vi "commander4.vi"() -> ()   [LabVIEW 2015]
uses:
  G_SEN.vi
  G_NAV.vi
  G_LCM.vi
  G_VEH.vi
  <vilib>/Analysis/Matrix/Numeric/Conversions/Array To Matrix - RA.vi
  <vilib>/Analysis/Matrix/Numeric/Conversions/Array To Matrix - RA2.vi
  <vilib>/Analysis/Matrix/Numeric/Multiply/Multiply - RM,RM.vi
  <vilib>/Analysis/Matrix/Numeric/Conversions/Matrix To Array - RM.vi
  G_PATH.vi
  G_DATA.vi
  <vilib>/Analysis/Matrix/NI_Matrix.lvlib
panel:
  in  "lpf gain":dbl=0.01 format="%#_13g"
  in  "KR":dbl
  in  "Kheading":dbl
  in  "Kdist":dbl
  out "String":string
  out "Taxi":dbl[](array[numeric])
  out "EURECAR_VISION":T1
  out "count":i32
  out "Array 3":picture[](array[picture])
  out "Array 2":picture[](array[picture])
  out "sign 2":picture[](array[picture])
  out "sign":picture[](array[picture])
  in  "TTL":bool
  out "STOP":bool
  out "go":bool
  in  "Steering gain":dbl=1.07
  in  "Steering LPF gain":dbl
  in  "vehicel width":dbl=2.1999999999999997
  out "obs shift":dbl=-0.0 format="%.2f"
  in  "lane keep":bool
  in  "vel":bool
  in  "replay":bool
  in  "lane":bool
  in  "x":dbl min=-5.0 max=5.0 step=1.0
  out "lane_shift":dbl
  in  "Shift LPF gain":dbl=0.95
  out "display":u32=20
  out "control":u32=10
  out "update":bool=TRUE
  in  "save lcm":bool
  out "LCM Recv Data":string="SDT_GPS_DATA\t550\rGGA_1\t275\rGGA_2\t275\rRMC_1\t275\rIBEO_2202_T\t686\rRMC_2\t275\rEYE_RAW_T\t549\rPOS_T\t5352\rPATH_T\t1373\rCAN_T\t5486\rCON_T\t5458\r"
  out "GPS DATA 2":T2={"type"="WAAS", "x_lcc"=-423.72650605501394, "y_lcc"=-797.2504532505071, "latdev"=0.92, "londev"=0.92, "sats"=11, "gps_l1_ranges"=0, "gps_l1_mask_ranges"=0, "gps_l2_mask_ranges"=0, "Heading"=152.5234544430902, "lon"=127.356186, "lat"=36.368267, "time"="01:10:55.0", "hgps"=151.67000000000002, "lag"=0.0, "MAP"="KAIST"} {"lag" format="%#_5g"; "hgps" format="%#_5g"; "lat" format="%#_11g"; "lon" format="%#_11g"; "Heading" format="%#_5g"; "latdev" format="%#_4g"; "londev" format="%#_4g"}
  in  "Obs":bool=TRUE
  in  "Log":bool
  out "path":u32=10
  out "sensor":u32=10 format="%02.0f"
  out "Speed limit":dbl=20.0
  out "collision":bool
  in  "Load WPT":bool
  in  "Max. Vel.":dbl=20.0 min=-5.0 max=120.0 step=5.0
  in  "RESET PATH":bool
  out "col":i16(graph)
  out "stop":bool
  in  "Reverse":bool
  in  "STOP":bool
  out "Waveform Chart 4":cluster{"auto":i16, "run":i16}(graph)={"auto"=1, "run"=0}
  out "Waveform Chart 3":T3(graph)={"Steer_input"=0.0, "Steer_output"=-2.5, "handle"=1.691462017818249}
  out "Waveform Chart 2":T4(graph)={"VS_des"=0.0, "VS_can"=30.952437500000002, "VS_des"=20.0}
  out "Heading":cluster{"Heading":dbl, "hgps":dbl}(graph)={"Heading"=152.5234544430902, "hgps"=151.67000000000002}
  out "XY Graph 2":cluster{"Y":dbl[], "Y":dbl[]}[](graph)=[{"Y"=[-423.72650605501394], "Y"=[-797.2504532505071]}, {"Y"=array[29568 elements], "Y"=array[29568 elements]}, {"Y"=array[29568 elements], "Y"=array[29568 elements]}, {"Y"=[-419.18788283563754], "Y"=[-805.7085038383482]}]
  out "Gauge":cluster{dbl, dbl, dbl}(knob)={0.0, 30.952437500000002, 20.0} scale=-20.0..140.0
  out "Meter":cluster{dbl, dbl, dbl}(knob)={0.0, -2.5, 1.691462017818249} scale=-550.0..550.0
  out "XY Graph":cluster{"Y":dbl[], "Y":dbl[]}[](graph)=[{"Y"=[0.0], "Y"=[0.0]}, {"Y"=array[500 elements], "Y"=array[500 elements]}, {"Y"=array[500 elements], "Y"=array[500 elements]}, {"Y"=[], "Y"=[]}, {"Y"=[-0.003264064170771075], "Y"=[-0.9807019516255565]}, {"Y"=[], "Y"=[]}, {"Y"=[0.0, 3.415667538320122e-05, 0.00013662669994118914, 0.00030741006844436924, 0.0005465067717977945, 0.0008539167977232864, 0.0012296401303046878, 0.0016736767499878624, 0.002186026633808069, 0.002766689755162588, 0.0034156660840380937, 0.004132955586555909, 0.0049185582258814975, 0.005772473960860225, 0.006694702747381598, 0.007685244537924518, 0.008744099280875162, 0.009871266920981725, 0.011066747400491295, 0.01233054065687611, 0.013662646624879926, 0.015063065235381146, 0.016531796415847566, 0.01806884008965426, 0.019674196177675185, 0.021347864596464206, 0.023089845258937203, 0.024900138075281575, 0.026778742951591994, 0.028725659789870406, 0.03074088848984502, 0.0328244289464692, 0.03497628105219519, 0.03719644469515515, 0.039484919760298, 0.04184170612916205, 0.044266803678965516, 0.046760212284425506, 0.04932193181639377, 0.05195196214162934, 0.05465030312393537, 0.05741695462347707, 0.06025191649655426, 0.06315518859628355, 0.06612677077237095, 0.06916666287065709, 0.07227486473311728, 0.07545137619899833, 0.07869619710345432, 0.08200932727800136, 0.0853907665511997, 0.08884051474774424, 0.09235857168846451, 0.0959449371912342, 0.09959961106960691, 0.1033225931346351, 0.10711388319305115, 0.11097348104817684, 0.11490138650015069, 0.11889759934479116, 0.12296211937541557, 0.12709494638102115, 0.1312960801474219, 0.13556552045656645, 0.1399032670874476, 0.14430931981473805, 0.1487836784101546, 0.15332634264177614, 0.15793731227381613, 0.16261658706753224, 0.167364166779862, 0.17218005116524182, 0.17706423997333331, 0.18201673295106957, 0.1870375298417457, 0.19212663038501887, 0.19728403431690822, 0.20250974137024969, 0.2078037512735591, 0.21316606375307856, 0.21859667853004794, 0.224095595323206, 0.22966281384742615, 0.23529833381371645, 0.24100215493058386, 0.2467742769013057, 0.25261469942756776, 0.25852342220582614, 0.2645004449300359, 0.2705457672900593, 0.27665938897257547, 0.2828413096606255, 0.28909152903361246, 0.29541004676730154, 0.3017968625342746, 0.3082519760032483, 0.31477538683952844, 0.3213670947045557, 0.3280270992572696, 0.3347554001516073, 0.3415519970390051], "Y"=[0.0, 0.2999999974073812, 0.5999999792590494, 0.8999999299992923, 1.1999998340723999, 1.4999996759226633, 1.7999994399943782, 2.0999991107318436, 2.399998672579363, 2.6999981099812467, 2.9999974073818105, 3.299996549225377, 3.5999955199562788, 3.899994304018856, 4.199992885857458, 4.4999912499164445, 4.79998938064019, 5.099987262473074, 5.399984879859496, 5.6999822172438686, 5.999979259070614, 6.299975989784169, 6.599972393828998, 6.899968455649568, 7.199964159690372, 7.49995949039592, 7.799954432210742, 8.099948969579385, 8.39994308694642, 8.69993676875644, 8.999929999454059, 9.299922763483913, 9.599915045290667, 9.899906829319006, 10.199898100013643, 10.499888841819322, 10.7998790391808, 11.099868676542881, 11.399857738350386, 11.699846209048172, 11.99983407308112, 12.299821314894148, 12.599807918932202, 12.899793869640266, 13.199779151463357, 13.49976374884652, 13.799747646234845, 14.099730828073453, 14.399713278807496, 14.699694982882185, 14.999675924742744, 15.299656088834453, 15.599635459602627, 15.89961402149262, 16.199591758949833, 16.499568656419704, 16.799544698347727, 17.09951986917942, 17.39949415336036, 17.699467535336172, 17.99943999955252, 18.299411530455117, 18.59938211248973, 18.899351730102172, 19.1993203677383, 19.49928800984403, 19.799254640865325, 20.099220245248205, 20.399184807438736, 20.69914831188305, 20.999110743027323, 21.29907208531778, 21.599032323200728, 21.898991441122508, 22.198949423529527, 22.498906254868253, 22.798861919585207, 23.098816402126975, 23.398769686940213, 23.698721758471617, 23.99867260116797, 24.2986221994761, 24.598570537842914, 24.898517600715373, 25.198463372540502, 25.498407837765416, 25.79835098083727, 26.09829278620331, 26.398233238310823, 26.698172321607203, 26.99811002053988, 27.29804631955638, 27.59798120310429, 27.897914655631272, 28.197846661585064, 28.497777205413485, 28.797706271564408, 29.097633844485816, 29.397559908625745, 29.69748444843231, 29.997407448353716]}, {"Y"=[0.10980542765272491, 0.10806044137247942, 0.10635032580737544, 0.104673921649975, 0.10303006959299141, 0.10141761032888227, 0.09983538455036242, 0.09828223294993985, 0.09675699622027753, 0.09525851505393765, 0.09378563014347793, 0.09233718218161399, 0.09091201186080297, 0.08950895987376092, 0.08812686691304447, 0.08676457367116494, 0.08542092084088723, 0.08409474911467027, 0.08278489918517548, 0.08149021174496349, 0.08020952748669616, 0.07894168710288615, 0.0776855312861918, 0.07643990072917548, 0.07520363612444933, 0.0739755781645722, 0.07275456754225837, 0.0715394449499672, 0.07032905108035967, 0.06912222662605058, 0.06791781227959523, 0.06671464873360664, 0.0655115766806996, 0.06430743681348358, 0.06310106982451921, 0.06189131640636622, 0.060677017251687365, 0.05945701305309389, 0.058230144503097575, 0.05699525229435495, 0.055751177119486156], "Y"=[0.6336267682406714, 1.1336410424573864, 1.6336557286203426, 2.133670813034119, 2.6336862820032167, 3.1337021218320134, 3.6337183188251365, 4.133734859286937, 4.6337517295219435, 5.133768915834733, 5.633786404529633, 6.133804181911268, 6.633822234284019, 7.133840547952512, 7.633859109221073, 8.133877904394181, 8.633896919776435, 9.13391614167234, 9.6339355563863, 10.133955150222762, 10.633974909486257, 11.133994820481387, 11.634014869512427, 12.134035042883955, 12.634055326900528, 13.134075707866467, 13.634096172086398, 14.13411670586483, 14.634137295506035, 15.13415792731482, 15.63417858759538, 16.134199262652274, 16.63421993879005, 17.134240602313263, 17.63426123952624, 18.134281836733553, 18.63430238023961, 19.134322856348966, 19.63434325136609, 20.134363551595385, 20.634383743341537]}, {"Y"=array[29568 elements], "Y"=array[29568 elements]}, {"Y"=array[500 elements], "Y"=array[500 elements]}, {"Y"=array[500 elements], "Y"=array[500 elements]}, {"Y"=[], "Y"=[]}, {"Y"=array[354 elements], "Y"=array[354 elements]}, {"Y"=array[4481 elements], "Y"=array[4481 elements]}, {"Y"=[-10.906571416296051, -10.659344379334508, -10.34492577533353, -9.93850331576459, -9.71566777130286, -9.617100686731023, -9.57320063609188, -9.426816486963638, -9.293613509628, -8.974678106104058, -7.209506291757908, -6.90626493691018, -6.814280811761357, -6.626676847115707, -6.119491263512161, -6.1059628797693914, -6.085673606595757, -6.071004517427587, -6.045215959436017, -5.462324651776553, -5.399808018833683, -5.381642021310995, -5.354978164273503, -5.351347300587539, -5.350759626886299, -1.948739875648812, 1.1635619052210888, 1.4000132038748632, 1.79606313236674, 1.872997152146425, 2.072930894516457, 2.2294377900724553, 2.304490671480748, 2.374735567627388, -8.627987914322672], "Y"=[32.45496234377471, 32.57681568932276, 32.50781451663184, 41.97530497964458, 30.70496770334178, 42.13780871287706, 31.0817543350392, 29.14220978725092, 42.297664351343066, 42.48410167536142, 44.71997382146028, 45.15583981418206, 24.809553609585002, 24.87733062282879, 24.546848844229835, 23.802254674654517, 23.07872875274249, 22.414456854385506, 21.752015731077318, 26.95016292110075, 24.89117948175122, 23.27716434297315, 21.834425288545347, 21.21173993871122, 22.46815793251327, 21.902985584007844, 33.75913455824824, 22.47395885729035, 35.4201133198724, 32.270336548658136, 22.361847591451152, 20.901773227911, 20.286851457563237, 19.711602445657494, 10.737594654789199]}, {"Y"=[-0.925, -0.925, -0.925, -0.6775, -0.6775, -0.925, -0.925, -0.925, -0.925, -0.6775, -0.6775, -0.925, -0.925, -0.925, 0.9025, 0.9025, 0.9025, 0.6775, 0.6775, 0.9025, 0.9025, 0.9025, 0.9025, 0.6775, 0.6775, 0.9025, 0.9025, 0.9025, -0.925], "Y"=[-0.75, -0.224, 0.224, 0.224, -0.224, -0.224, 0.224, 2.415, 2.885, 2.885, 2.415, 2.415, 2.885, 3.5, 3.5, 2.885, 2.415, 2.415, 2.885, 2.885, 2.415, 0.224, -0.224, -0.224, 0.224, 0.224, -0.224, -0.75, -0.75]}, {"Y"=[-1.989725401977954], "Y"=[16.427453516317758]}]
  in  "Make WPT":bool
  out "left":bool
  # "V2I Traffic Signal"
  # "CNN\nSign\nDetection"
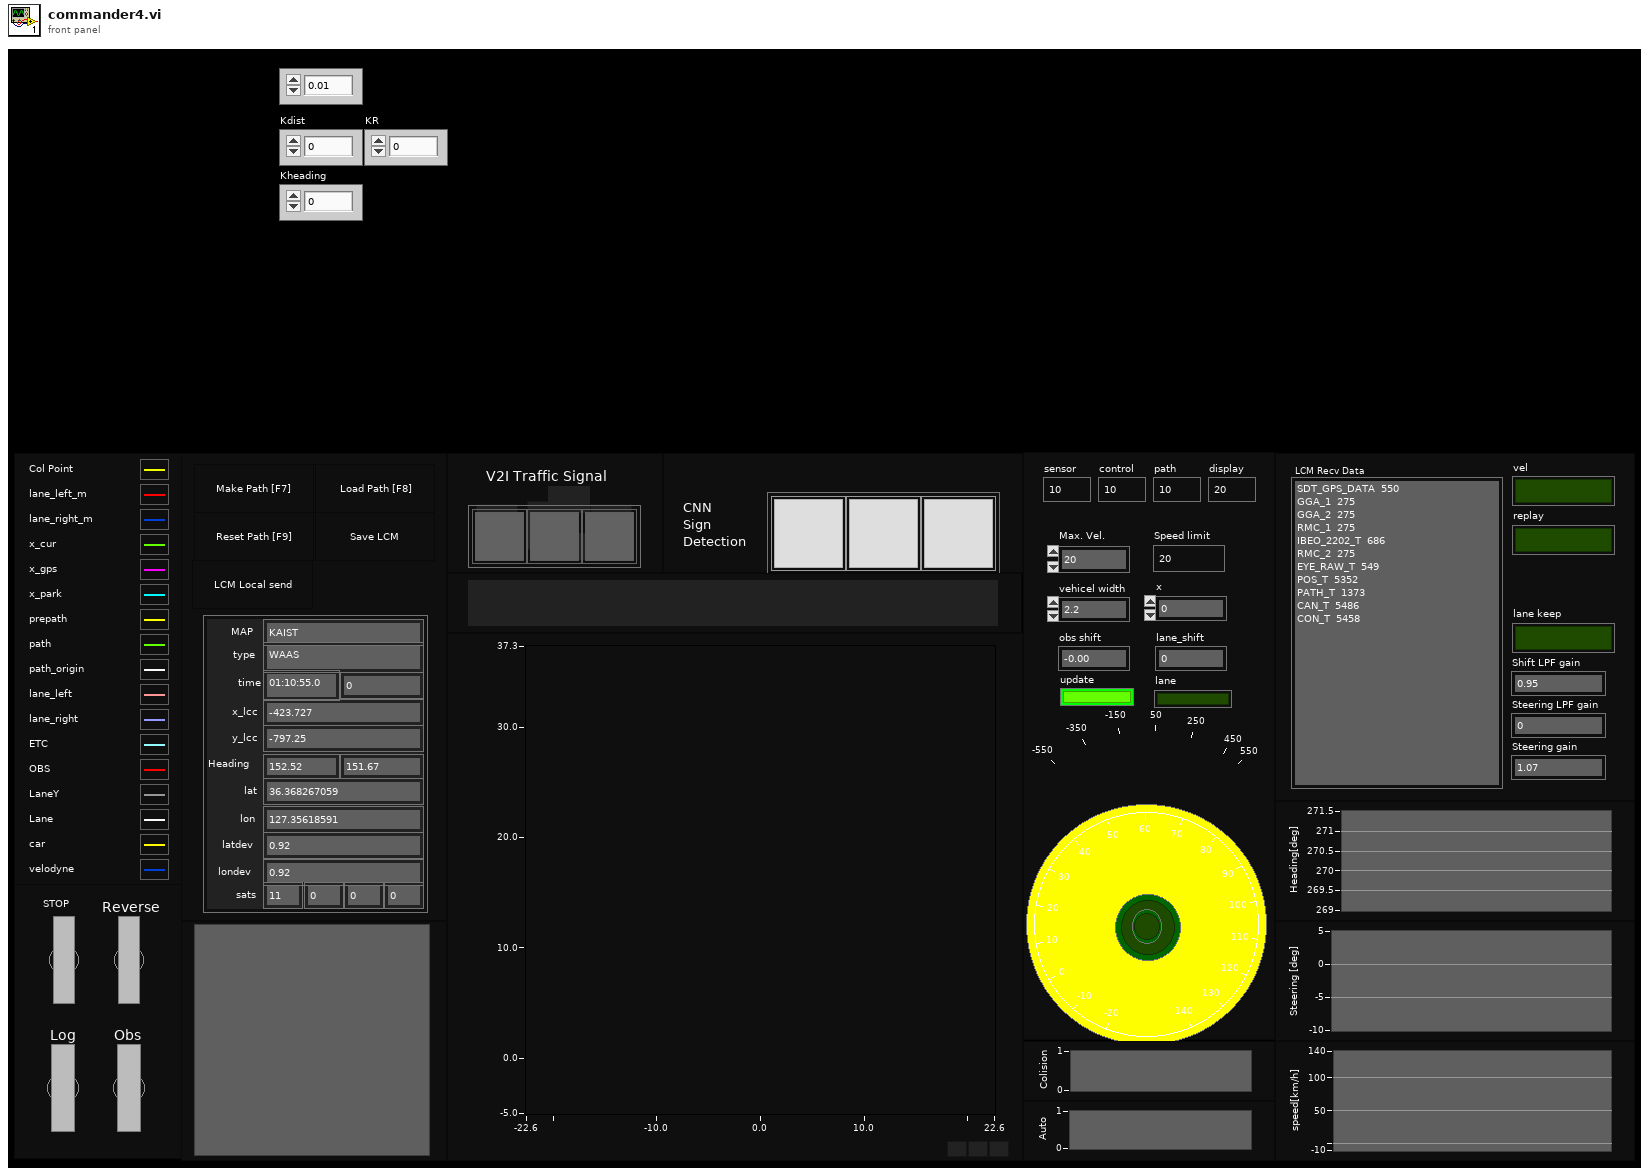
[diagram p1: front panel]
types:
  T1 = cluster{"hash":i64, "sys time":i64, "status":i32, "TS_num":i32, "TS_type":i32[], "TS_loc_x":dbl[], "TS_loc_y":dbl[]}
  T2 = cluster{"type":string, "x_lcc":dbl, "y_lcc":dbl, "latdev":sgl, "londev":sgl, "sats":u8, "gps_l1_ranges":u8, "gps_l1_mask_ranges":u8, "gps_l2_mask_ranges":u8, "Heading":dbl, "lon":sgl, "lat":sgl, "time":string, "hgps":dbl, "lag":dbl, "MAP":string}
  T3 = cluster{"Steer_input":dbl, "Steer_output":dbl, "handle":dbl}
  T4 = cluster{"VS_des":dbl, "VS_can":dbl, "VS_des":dbl}
  T5 = enum8{"Enabled", "Disabled", "Disabled and Grayed Out"}
  T6 = cluster{"X":cluster{"idx":i32, "x":dbl, "y":dbl, "h":dbl, "x_path":dbl}}[]
  T7 = cluster{"idx":i32, "x":dbl, "y":dbl, "h":dbl, "x_path":dbl}
  T8 = cluster{"idx":i32, "x":dbl, "y":dbl, "hp":dbl, "x_path":dbl}
  T9 = cluster{"GPSTime":dbl, "attitude[2]":dbl, "lcc[0]":dbl, "lcc[1]":dbl, "heading_GPS":dbl}
  T10 = cluster{"Steer_input":dbl, "Steer_output":dbl, "VS_des":dbl, "VS_can":dbl, "heading":dbl, "auto":bool, "run":bool, "x":dbl, "y":dbl}
  T11 = cluster{"hash":i64, "sys time":i64, "s_lat":dbl, "s_lon":dbl, "d_lat":dbl, "d_lon":dbl, "Message":i64}
  T12 = typedef "imagedata.ctl" = cluster{"image type":i32, "image depth":i32, "image":u8[], "mask":u8[], "colors":u32[], "Rectangle":cluster{"left":i16, "top":i16, "right":i16, "bottom":i16}}
  T13 = typedef "NI_Matrix.lvlib/RealMatrix.ctl" = dbl[][]
  T14 = cluster{"Minimum":dbl, "Minimum":dbl, "Minimum":dbl, "Minimum":dbl, "Minimum":dbl}
  T15 = cluster{"X":cluster{"c_idx":i32, "xc":dbl, "yc":dbl, "hc":dbl, "xc_path":dbl}}[]
  T16 = cluster{"hash":i64, "sys time":i64, "time":dbl, "x":dbl, "y":dbl, "h":dbl, "numSV":i32, "postype":i32, "lag":i32, "hordev":dbl, "lat":dbl, "lon":dbl, "hgt":dbl, "map_idx":i32}
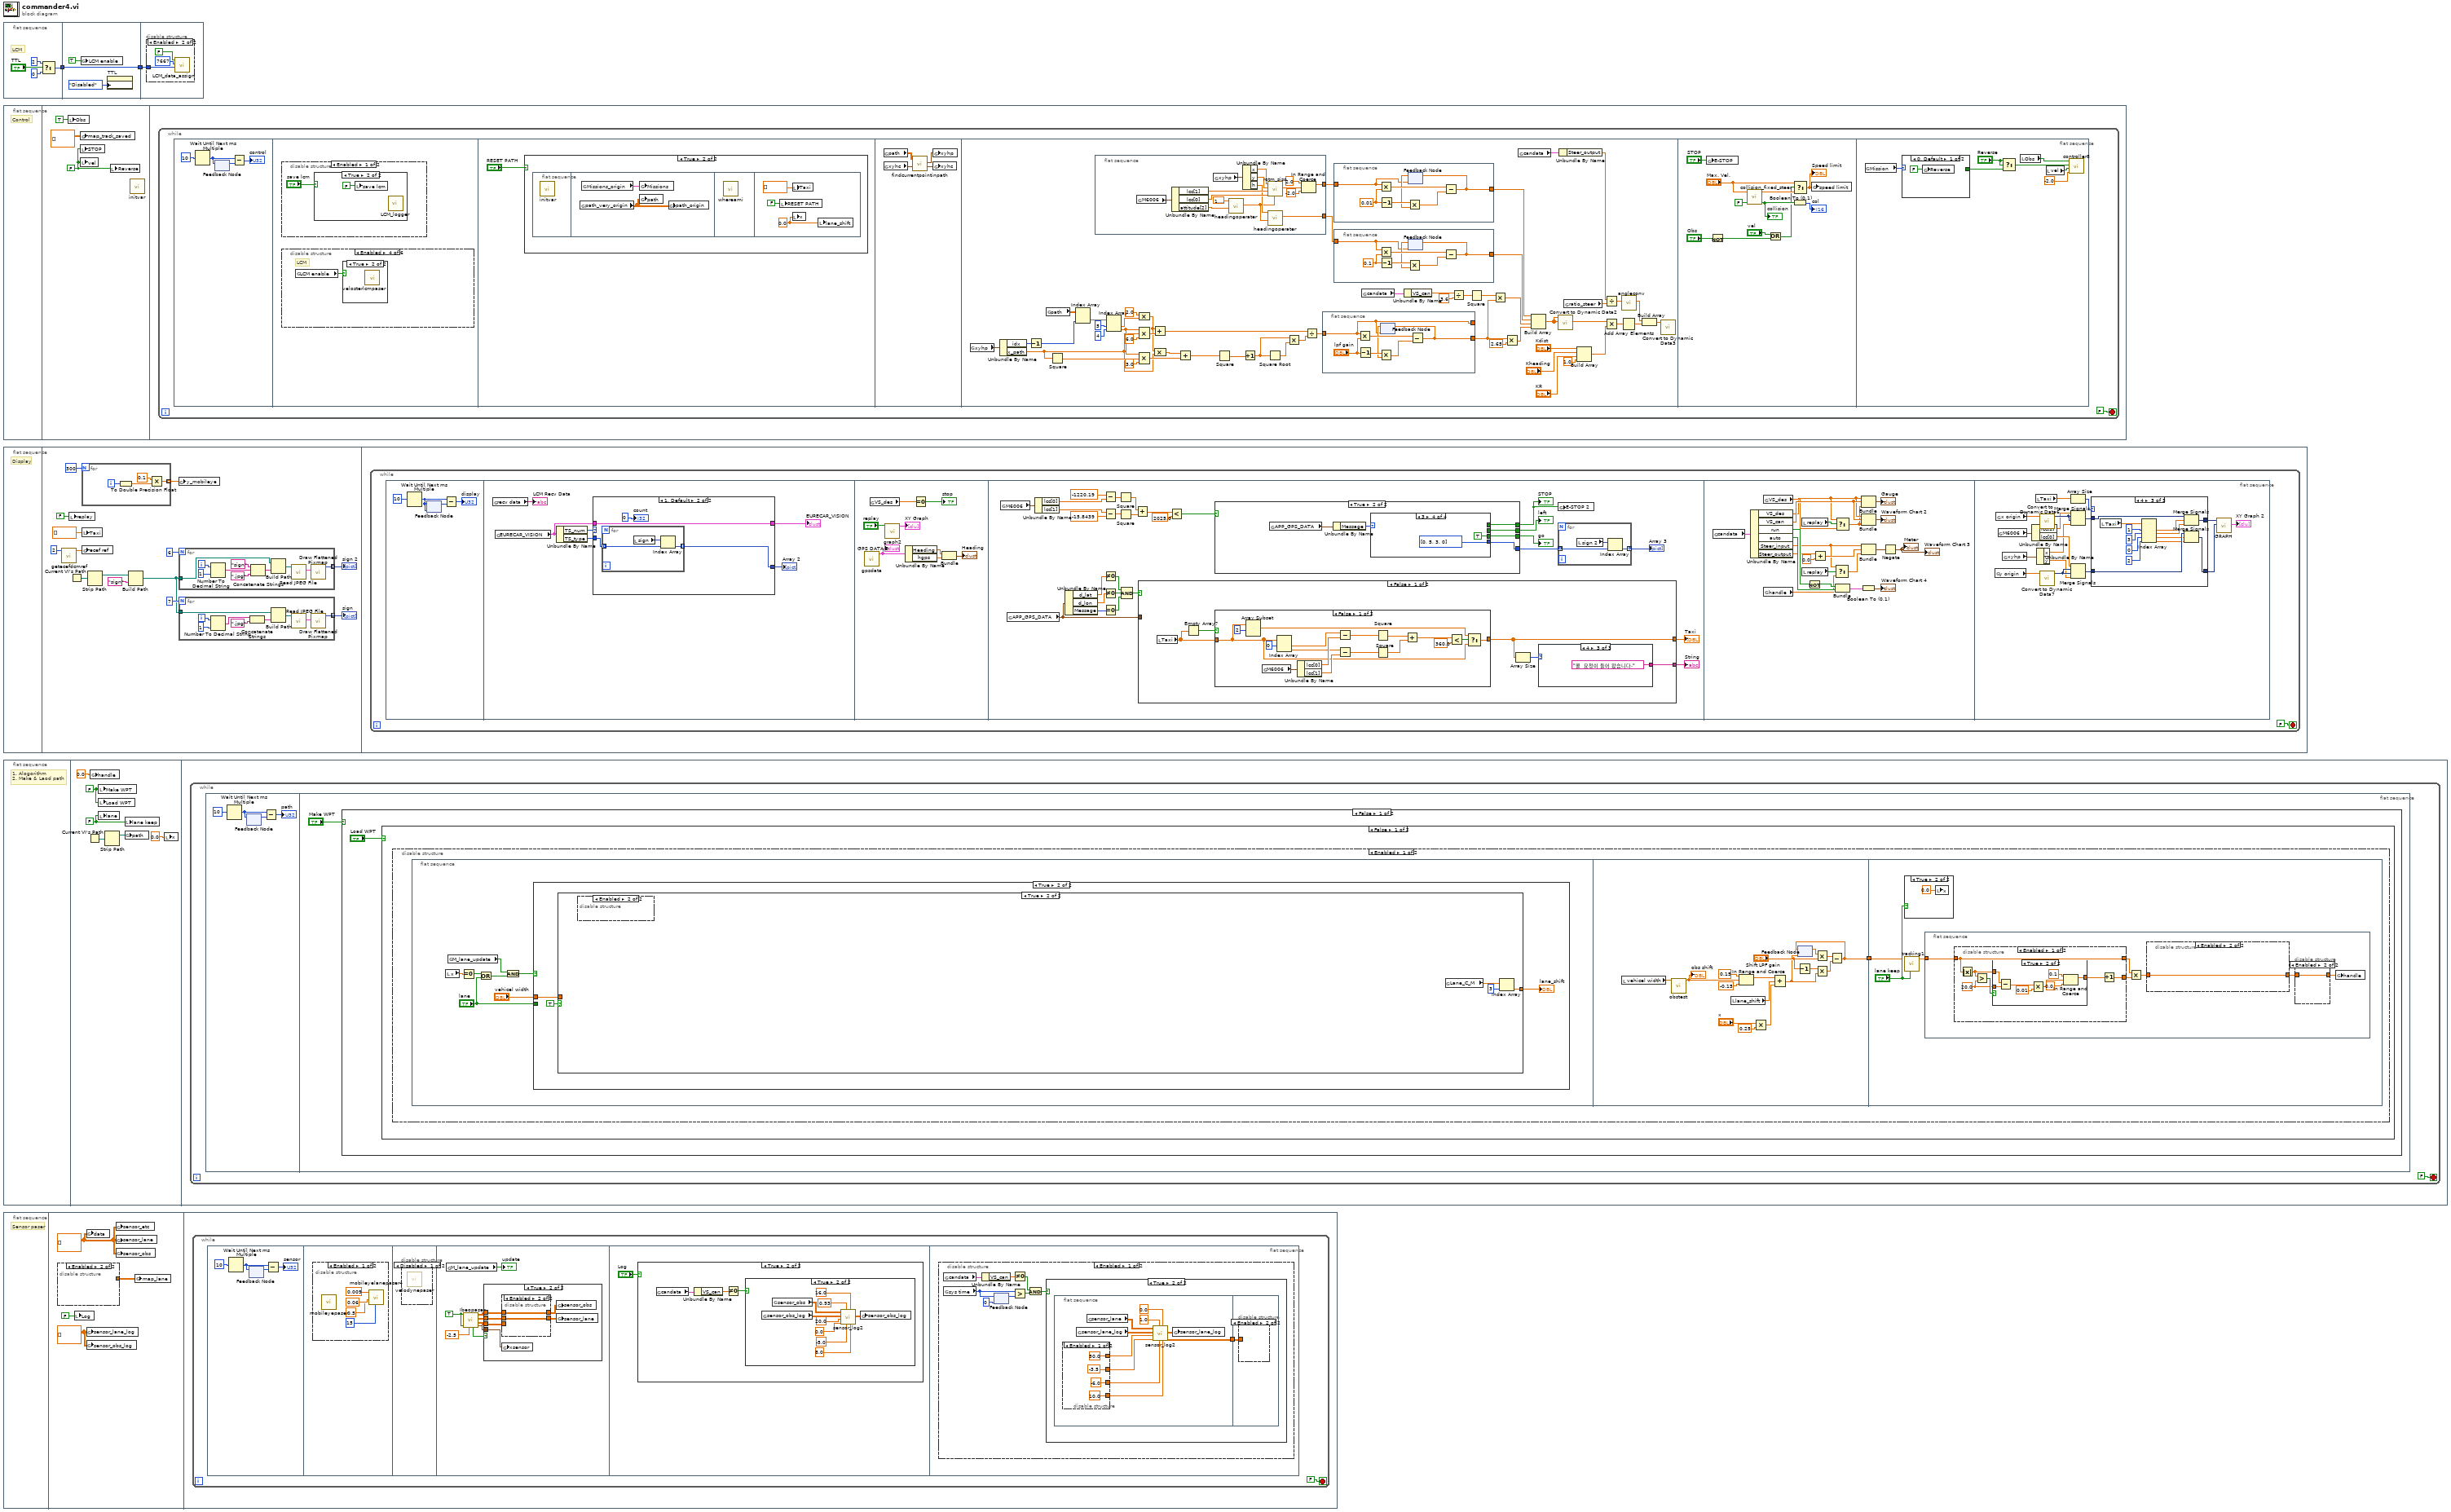
[diagram p0: block diagram]
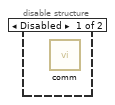
[diagram p2: hidden frame]
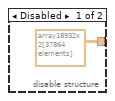
[diagram p3: hidden frame]
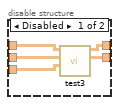
[diagram p7: hidden frame]
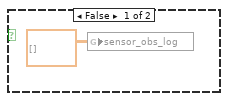
[diagram p8: hidden frame]
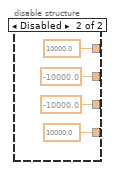
[diagram p11: hidden frame]
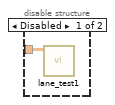
[diagram p12: hidden frame]
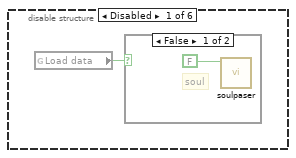
[diagram p16: hidden frame]
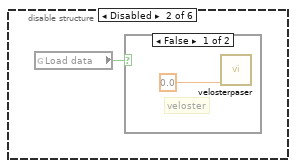
[diagram p18: hidden frame]
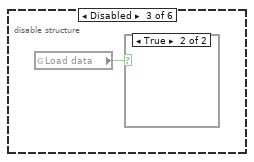
[diagram p20: hidden frame]
diagram:
  n1 = flat-sequence {
    tunnel: [w3] -> w1
    tunnel: [w8] -> w2
    tunnel: w1 -> [w8]
    tunnel: w2 -> [w10]
    frame #0 {
      # "LCM"
      n2 = Select(t=u16 2 ("time-to-live"), s="TTL", f=u16 0 ("time-to-live")) -> (s? t:f=w3:u16)
    }
    frame #1 {
      n3 = global write "G_LCM.vi" "LCM enable"(TRUE ("x")) -> ()
      n4 = property on="TTL" class="Bool (strict)"("DisabledEnum"=T5."Disabled" ("Disabled")) -> ()  [unwired: 2 in, 2 out]
    }
    frame #2 {
      n5 = disable-structure shown="Enabled" {
        disable-tunnel: w10 -> [_ w11]
        frame Disabled {
          n6 = call "comm.vi"() -> ()  [unwired: 12 in]
        }
        frame Enabled {
          n7 = call "LCM_data_assign.vi"("time-to-live"=w11, "port"=u16 7667, "velodyne enable"=FALSE) -> ()  [unwired: 9 in]
        }
      }
    }
  }
  n8 = flat-sequence {
    frame #0 {
      # "Control"
    }
    frame #1 {
      w15 = FALSE ("LCM")
      n9 = local write "Obs"(TRUE ("obs")) -> ()
      n10 = global write "G_PATH.vi" "map_track_saved"(dbl[][] [] ("map_track_saved")) -> ()
      n11 = local write "STOP"(w15) -> ()
      n12 = local write "vel"(w15) -> ()
      n13 = local write "Reverse"(w15) -> ()
      n14 = call "initvar.vi"() -> ()  [unwired: 12 in]
    }
    frame #2 {
      n15 = while {
        stop <- FALSE ("Boolean") stop-if-true
        n16 = flat-sequence {
          frame #0 {
            n17 = Wait Until Next ms Multiple(millisecond multiple=u32 10 ("milliseconds to wait")) -> (millisecond timer value=w18:u32)
            n18 = feedback #1() -> (w19:u32)  [unwired: 1 in]
            n19 = feedback-in #1(w18) -> ()
            n20 = Subtract(x=w18, y=w19) -> (x-y=→"control":u32)
          }
          frame #1 {
            n21 = disable-structure shown="Enabled" {
              frame Enabled {
                n22 = case shown="True" "save lcm" {
                  frame False {
                  }
                  frame True {
                    n23 = local write "save lcm"(FALSE ("save lcm")) -> ()
                    n24 = call "LCM_logger.vi"() -> ()  [unwired: 12 in]
                  }
                }
              }
              frame Disabled {
              }
            }
            n25 = disable-structure shown="Enabled" {
              frame Disabled {
                n26 = global read "G_DATA.vi" "Load data"() -> (w24:bool)
                n27 = case shown="False" w24 {
                  frame False {
                    # "soul"
                    n28 = call "soulpaser.vi"("rionav?"=FALSE) -> ()  [unwired: 11 in]
                  }
                  frame True {
                  }
                }
              }
              frame Disabled {
                n29 = global read "G_DATA.vi" "Load data"() -> (w26:bool)
                n30 = case shown="False" w26 {
                  frame False {
                    # "veloster"
                    n31 = call "velosterpaser.vi"("x"=0.0) -> ()  [unwired: 11 in]
                  }
                  frame True {
                  }
                }
              }
              frame Disabled {
                n32 = global read "G_DATA.vi" "Load data"() -> (w28:bool)
                n33 = case shown="True" w28 {
                  frame False {
                    # "webot"
                    n34 = call "webot.vi"() -> ()  [unwired: 12 in]
                  }
                  frame True {
                  }
                }
              }
              frame Enabled {
                # "LCM"
                n35 = global read "G_LCM.vi" "LCM enable"() -> (w29:bool)
                n36 = case shown="True" w29 {
                  frame False {
                  }
                  frame True {
                    n37 = call "velosterlcmpaser.vi"() -> ()  [unwired: 11 in, 1 out]
                  }
                }
              }
              frame Disabled {
              }
              frame Disabled {
                # "RCcar"
                n38 = global read "G_DATA.vi" "Load data"() -> (w30:bool)
                n39 = case shown="True" w30 {
                  frame False {
                  }
                  frame True {
                    n40 = global read "G_VEH.vi" "VS_des"() -> (w31:dbl)
                    n41 = global read "G_VEH.vi" "handle"() -> (w32:dbl)
                    n42 = shared-variable "NI-sbRIO9606-01866155\\sharedvari.lvlib\\vs_des"(w31) -> ()  [unwired: 1 in, 1 out]
                    n43 = shared-variable "NI-sbRIO9606-01866155\\sharedvari.lvlib\\steer_input"(w32) -> ()  [unwired: 1 in, 1 out]
                  }
                }
              }
            }
          }
          frame #2 {
            n44 = case shown="True" "RESET PATH" {
              frame False {
              }
              frame True {
                n45 = flat-sequence {
                  frame #0 {
                    n46 = call "initvar.vi"() -> ()  [unwired: 12 in]
                  }
                  frame #1 {
                    n47 = global read "G_PATH.vi" "path_very_origin"() -> (w35:dbl[][])
                    n48 = global read "G_PATH.vi" "Missions_origin"() -> (w34:T6)
                    n49 = global write "G_PATH.vi" "Missions"(w34) -> ()
                    n50 = global write "G_PATH.vi" "path"(w35) -> ()
                    n51 = global write "G_PATH.vi" "path_origin"(w35) -> ()
                  }
                  frame #2 {
                    n52 = call "whereami.vi"() -> ()  [unwired: 12 in]
                  }
                  frame #3 {
                    w37 = 0.0 ("x")
                    n53 = local write "RESET PATH"(FALSE ("RESET PATH")) -> ()
                    n54 = local write "Taxi"(dbl[] [] ("Taxi")) -> ()
                    n55 = local write "x"(w37) -> ()
                    n56 = local write "lane_shift"(w37) -> ()
                  }
                }
              }
            }
          }
          frame #3 {
            n57 = global read "G_PATH.vi" "path"() -> (w41:dbl[][])
            n58 = global read "G_VEH.vi" "xyhc"() -> (w40:T7)
            n59 = call "findcurrentpointinpath.vi"("xyhc_in"=w40, "path_updated"=w41) -> ("xyhc_out"=w42:T7, "xyhp"=w39:T8)  [unwired: 8 in]
            n60 = global write "G_VEH.vi" "xyhp"(w39) -> ()
            n61 = global write "G_VEH.vi" "xyhc"(w42) -> ()
          }
          frame #4 {
            n62 = global read "G_VEH.vi" "xyhp"() -> (w94:T7)
            n63 = Unbundle By Name(w94) -> ("idx"=w93:i32, "x_path"=w78:dbl)
            n64 = Decrement(x=w93) -> (x-1=w91:i32)
            n65 = global read "G_PATH.vi" "path"() -> (w92:dbl[][])
            n66 = Square(x=w78) -> (x^2=w83:dbl)
            n67 = Index Array(array=w92, index (col)=w91) -> (element=w90:dbl[])  [unwired: 1 in]
            n68 = flat-sequence {
              tunnel: [w106] -> w58
              tunnel: [w102] -> w60
              frame #0 {
                n69 = global read "G_NAV.vi" "M6006"() -> (w109:T9)
                n70 = Unbundle By Name(w109) -> ("lcc[1]"=w111:dbl, "lcc[0]"=w112:dbl, "attitude[2]"=w114:dbl)
                n71 = global read "G_VEH.vi" "xyhp"() -> (w110:T7)
                n72 = call "headingoperater.vi"("h1"=w114, "h2"=1.5707963267948966) -> ("h2-h1"=w107:dbl)  [unwired: 8 in, 1 out]
                n73 = Unbundle By Name(w110) -> ("x"=w115:dbl, "y"=w116:dbl, "h"=w108:dbl)
                n74 = call "rotm_siso.vi"("angle[rad]"=w107, "y0"=w112, "x0"=w111, "y"=w116, "x"=w115) -> ("y'"=w103:dbl)  [unwired: 5 in, 1 out]
                n75 = call "headingoperater.vi"("h1"=w107, "h2"=w108) -> ("h2-h1"=w106:dbl)  [unwired: 8 in, 1 out]
                n76 = In Range and Coerce(upper limit=2.0, x=w103, lower limit=-2.0) -> (coerced(x)=w102:dbl)  [unwired: 1 out]
              }
            }
            n77 = Index Array(array=w90, index #1=5 ("index"), index #2=4 ("index")) -> (element #1=w85:dbl, element #2=w82:dbl)
            n78 = Compound Arithmetic op=MULTIPLY(2.0 ("value"), w85) -> (w79:dbl)
            n79 = Compound Arithmetic op=MULTIPLY(w82, w78, 6.0 ("value")) -> (w86:dbl)
            n80 = Compound Arithmetic op=MULTIPLY(w82, w83, 3.0 ("value")) -> (w80:dbl)
            n81 = Add(x=w79, y=w86) -> (x+y=w72:dbl)
            n82 = Compound Arithmetic op=MULTIPLY(w79, w78) -> (w77:dbl)
            n83 = Add(x=w77, y=w80) -> (x+y=w76:dbl)
            n84 = Square(x=w76) -> (x^2=w75:dbl)
            n85 = Increment(x=w75) -> (x+1=w73:dbl)
            n86 = Square Root(x=w73) -> (sqrt(x)=w74:dbl)
            n87 = Multiply(x=w73, y=w74) -> (x*y=w63:dbl)
            n88 = Divide(x=w72, y=w63) -> (x/y=w62:dbl)
            n89 = flat-sequence {
              tunnel: w62 -> [w124]
              tunnel: [w125] -> w61
              tunnel: [w124] -> _
              frame #0 {
                n90 = Multiply(x=w124, y="lpf gain") -> (x*y=w130:dbl)
                n91 = Decrement(x="lpf gain") -> (x-1=w128:dbl)
                n92 = feedback #2(w124) -> (w127:dbl)
                n93 = Multiply(x=w128, y=w127) -> (x*y=w126:dbl)
                n94 = Subtract(x=w130, y=w126) -> (x-y=w125:dbl)
                n95 = feedback-in #2(w125) -> ()
              }
            }
            n96 = flat-sequence {
              tunnel: w60 -> [w118]
              tunnel: [w117] -> w59
              frame #0 {
                w122 = 0.01 ("lpf gain")
                n97 = Multiply(x=w118, y=w122) -> (x*y=w123:dbl)
                n98 = Decrement(x=w122) -> (x-1=w121:dbl)
                n99 = feedback #3(w118) -> (w120:dbl)
                n100 = Multiply(x=w121, y=w120) -> (x*y=w119:dbl)
                n101 = Subtract(x=w123, y=w119) -> (x-y=w117:dbl)
                n102 = feedback-in #3(w117) -> ()
              }
            }
            n103 = flat-sequence {
              tunnel: [w96] -> w57
              tunnel: w58 -> [w95]
              frame #0 {
                w100 = 0.1 ("lpf gain 2")
                n104 = Multiply(x=w95, y=w100) -> (x*y=w101:dbl)
                n105 = Decrement(x=w100) -> (x-1=w99:dbl)
                n106 = feedback #4(w95) -> (w98:dbl)
                n107 = Multiply(x=w99, y=w98) -> (x*y=w97:dbl)
                n108 = Subtract(x=w101, y=w97) -> (x-y=w96:dbl)
                n109 = feedback-in #4(w96) -> ()
              }
            }
            n110 = global read "G_VEH.vi" "candata"() -> (w71:T10)
            n111 = Unbundle By Name(w71) -> ("VS_can"=w70:dbl)
            n112 = Divide(x=w70, y=3.6) -> (x/y=w68:dbl)
            n113 = Square(x=w68) -> (x^2=w67:dbl)
            n114 = Multiply(x=w67, y=w61) -> (x*y=w66:dbl)
            n115 = Multiply(x=w61, y=2.65) -> (x*y=w64:dbl)
            n116 = global read "G_VEH.vi" "candata"() -> (w49:T10)
            n117 = Build Array(w59, w57, w66, w64) -> (w51:dbl[])
            n118 = call "Convert to Dynamic Data2"("Array"=w51) -> ()  [unwired: 3 in, 1 out]
            n119 = Unbundle By Name(w49) -> ("Steer_output"=w48:dbl)
            n120 = global read "G_VEH.vi" "ratio_steer"() -> (w47:dbl)
            n121 = Build Array("Kdist", "Kheading", "KR", 1.0 ("element")) -> (w52:dbl[])
            n122 = Divide(x=w48, y=w47) -> (x/y=w46:dbl)
            n123 = Multiply(x=w51, y=w52) -> (x*y=w50:dbl[])
            n124 = Add Array Elements(numeric array=w50) -> (sum=w45:dbl)
            n125 = call "angleconv.vi"("deg"=w46) -> ("rad"=w43:dbl)  [unwired: 9 in, 1 out]
            n126 = Build Array(w43, w45) -> (w44:dbl[])
            n127 = call "Convert to Dynamic Data3"("Array"=w44) -> ()  [unwired: 3 in, 1 out]
          }
          frame #5 {
            n128 = global write "G_VEH.vi" "E-STOP"("STOP") -> ()
            n129 = Not(x="Obs") -> (.not. x?=w133:bool)
            n130 = call "collision_fixed_steer.vi"("obsclose"=FALSE, "Max. Vel."="Max. Vel.") -> ("collision"=w141:bool, "speed limit"=w136:dbl)  [unwired: 8 in]
            "collision" <- w141
            n131 = Or(x="vel", y=w133) -> (x .or. y?=w131:bool)
            n132 = Boolean To (0,1)(Boolean=w141) -> (0, 1=→"col":i16)
            n133 = Select(t="Max. Vel.", s=w131, f=w136) -> (s? t:f=w135:dbl)
            "Speed limit" <- w135
            n134 = global write "G_VEH.vi" "speed limit"(w135) -> ()
          }
          frame #6 {
            n135 = global read "G_PATH.vi" "Mission"() -> (w144:i32)
            n136 = case shown="0, Default" w144 {
              tunnel: [_ w150] -> w147
              frame 0, Default {
                n137 = global write "G_VEH.vi" "Reverse"(FALSE ("Reverse")) -> ()
              }
              frame 9 {
                n138 = global read "G_VEH.vi" "Reverse"() -> (w150:bool)
              }
            }
            n139 = Select(t="Reverse", s="Reverse", f=w147) -> (s? t:f=w146:bool)
            n140 = local read "Obs"() -> (w143:bool)
            n141 = local read "vel"() -> (w142:bool)
            n142 = call "controller8.vi"("Neg max speed"=-2.0, "vel"=w142, "reverse"=w146, "obs"=w143) -> ()  [unwired: 8 in]
          }
        }
      }
    }
  }
  n143 = flat-sequence {
    frame #0 {
      # "Display"
    }
    frame #1 {
      n144 = call "getecefdcmref.vi"("map"=2) -> ("XYZ"=w152:dbl[])  [unwired: 10 in, 4 out]
      n145 = local write "replay"(FALSE ("replay")) -> ()
      n146 = Current VI's Path() -> (path=w161:path)
      n147 = for {
        N: 300 -> [_]
        tunnel: [w184] -> w164 mode=indexing
        i -> [w187]
        n148 = To Double Precision Float(number=w187) -> (double precision float=w186:dbl)
        n149 = Multiply(x=0.1, y=w186) -> (x*y=w184:dbl)
      }
      n150 = local write "Taxi"(dbl[] [] ("Taxi")) -> ()
      n151 = global write "G_NAV.vi" "ecef ref"(w152) -> ()
      n152 = Strip Path(path=w161) -> (stripped path=w160:path)  [unwired: 1 out]
      n153 = Build Path(base path=w160, name or relative path="sign") -> (appended path=w154:path)
      n154 = global write "G_SEN.vi" "y_mobileye"(w164) -> ()
      n155 = for {
        N: 6 -> [_]
        tunnel: [w173] -> w156 mode=indexing
        tunnel: w154 -> [w168]
        i -> [w172]
        n156 = Number To Decimal String(number=w172, width (-)=i16 1) -> (decimal integer string=w170:string)
        n157 = Concatenate Strings("sign" ("string"), w170, ".jpg") -> (w167:string)
        n158 = Build Path(base path=w168, name or relative path=w167) -> (appended path=w166:path)
        n159 = call <vilib>:"Read JPEG File.vi"("path to JPEG file"=w166) -> ("image data"=w174:T12)  [unwired: 8 in, 2 out]
        n160 = call <vilib>:"Draw Flattened Pixmap.vi"("image data"=w174) -> ("new picture"=w173:picture)  [unwired: 8 in]
      }
      "sign 2" <- w156
      n161 = for {
        N: 7 -> [_]
        tunnel: [w182] -> w157 mode=indexing
        tunnel: w154 -> [w177]
        i -> [w181]
        n162 = Number To Decimal String(number=w181, width (-)=i16 1) -> (decimal integer string=w179:string)
        n163 = Concatenate Strings(w179, ".jpg") -> (w176:string)
        n164 = Build Path(base path=w177, name or relative path=w176) -> (appended path=w175:path)
        n165 = call <vilib>:"Read JPEG File.vi"("path to JPEG file"=w175) -> ("image data"=w183:T12)  [unwired: 8 in, 2 out]
        n166 = call <vilib>:"Draw Flattened Pixmap.vi"("image data"=w183) -> ("new picture"=w182:picture)  [unwired: 8 in]
      }
      "sign" <- w157
    }
    frame #2 {
      n167 = while {
        stop <- FALSE ("exit") stop-if-true
        n168 = flat-sequence {
          frame #0 {
            n169 = Wait Until Next ms Multiple(millisecond multiple=u32 10 ("milliseconds to wait")) -> (millisecond timer value=w189:u32)
            n170 = feedback #5(w189) -> (w191:u32)
            n171 = feedback-in #5(w189) -> ()
            n172 = Subtract(x=w189, y=w191) -> (x-y=→"display":u32)
          }
          frame #1 {
            n173 = global read "G_LCM.vi" "recv data"() -> (→"LCM Recv Data":string)
            n174 = global read "G_LCM.vi" "EURECAR_VISION"() -> (w194:T1)
            n175 = Unbundle By Name(w194) -> ("TS_num"=w197:i32, "TS_type"=w196:i32[])
            n176 = case shown="1, Default" w197 {
              tunnel: w196 -> [_ w213]
              tunnel: [w206 w212] -> w195
              tunnel: w194 -> [_ w210]
              tunnel: [w199 w210] -> w193
              frame 0 {
                w208 = 100 ("x")
                n177 = local read "count"() -> (w209:i32)
                n178 = Increment(x=w209) -> (x+1=w204:i32)
                n179 = Max & Min(x=w208, y=w204) -> (min(x,y)=w203:i32)  [unwired: 1 out]
                n180 = local read "EURECAR_VISION"() -> (w200:T1)
                n181 = local write "count"(w203) -> ()
                n182 = Equal?(x=w208, y=w203) -> (x = y?=w202:bool)
                n183 = local read "Array 2"() -> (w205:picture[])
                n184 = Select(t=T1 {"hash"=0, "sys time"=0, "status"=0, "TS_num"=0, "TS_type"=[], "TS_loc_x"=[], "TS_loc_y"=[]} ("EURECAR_VISION"), s=w202, f=w200) -> (s? t:f=w199:T1)
                n185 = Select(t=picture[] [], s=w202, f=w205) -> (s? t:f=w206:picture[])
              }
              frame 1, Default {
                n186 = for {
                  tunnel: w213 -> [w215] mode=indexing
                  tunnel: [w214] -> w212 mode=indexing
                  n187 = local read "sign"() -> (w216:picture[])
                  n188 = Index Array(array=w216, index=w215) -> (element=w214:picture)
                }
                "count" <- 0 ("Numeric Control")
              }
            }
            "Array 2" <- w195
            "EURECAR_VISION" <- w193
          }
          frame #2 {
            n189 = call "gpsdata.vi"() -> ("GPS DATA 2"=w222:T2)  [unwired: 11 in]
            "GPS DATA 2" <- w222
            n190 = global read "G_VEH.vi" "VS_des"() -> (w218:dbl)
            n191 = call "graph2.vi"("replay"="replay") -> ("XY Graph"=→"XY Graph":cluster{"Y":dbl[], "Y":dbl[]}[])  [unwired: 9 in, 1 out]
            n192 = Unbundle By Name(w222) -> ("Heading"=w224:dbl, "hgps"=w223:dbl)
            n193 = Equal To 0?(x=w218) -> (x = 0?=→"stop":bool)
            n194 = Bundle("Heading"=w224, "hgps"=w223) -> (→"Heading":cluster{"Heading":dbl, "hgps":dbl})  [unwired: 1 in]
          }
          frame #3 {
            n195 = global read "G_NAV.vi" "M6006"() -> (w248:T9)
            n196 = global read "G_LCM.vi" "APP_GPS_DATA"() -> (w227:T11)
            n197 = Unbundle By Name(w248) -> ("lcc[0]"=w247:dbl, "lcc[1]"=w245:dbl)
            n198 = Unbundle By Name(w227) -> ("d_lat"=w232:dbl, "d_lon"=w233:dbl, "Message"=w234:i64)
            n199 = Subtract(x=-1220.19, y=w247) -> (x-y=w243:dbl)
            n200 = Subtract(x=w245, y=-15.8439) -> (x-y=w242:dbl)
            n201 = Not Equal To 0?(x=w232) -> (x != 0?=w231:bool)
            n202 = Not Equal To 0?(x=w233) -> (x != 0?=w230:bool)
            n203 = Equal To 0?(x=w234) -> (x = 0?=w229:bool)
            n204 = Square(x=w243) -> (x^2=w241:dbl)
            n205 = Square(x=w242) -> (x^2=w240:dbl)
            n206 = Compound Arithmetic op=AND(w231, w230, w229) -> (w228:bool)
            n207 = Add(x=w241, y=w240) -> (x+y=w239:dbl)
            n208 = case shown="False" w228 {
              tunnel: w227 -> [_ w283]
              tunnel: [w254 w278] -> w226
              tunnel: [w252 _] -> w225
              frame False {
                n209 = local read "Taxi"() -> (w256:dbl[])
                n210 = Empty Array?(array=w256) -> (empty?=w255:bool)
                n211 = case shown="False" w255 {
                  tunnel: w256 -> [w263 _]
                  tunnel: [w260 _] -> w254
                  frame False {
                    n212 = Array Subset(array=w263, index=2) -> (w261:dbl[])  [unwired: 1 in]
                    n213 = global read "G_NAV.vi" "M6006"() -> (w275:T9)
                    n214 = Index Array(array=w263, index #1=0 ("index")) -> (element #1=w270:dbl, element #2=w268:dbl)  [unwired: 1 in]
                    n215 = Unbundle By Name(w275) -> ("lcc[0]"=w269:dbl, "lcc[1]"=w267:dbl)
                    n216 = Subtract(x=w270, y=w269) -> (x-y=w271:dbl)
                    n217 = Subtract(x=w268, y=w267) -> (x-y=w272:dbl)
                    n218 = Square(x=w271) -> (x^2=w273:dbl)
                    n219 = Square(x=w272) -> (x^2=w274:dbl)
                    n220 = Add(x=w273, y=w274) -> (x+y=w265:dbl)
                    n221 = Less?(x=w265, y=360.0) -> (x < y?=w264:bool)
                    n222 = Select(t=w261, s=w264, f=w263) -> (s? t:f=w260:dbl[])
                  }
                  frame True {
                  }
                }
                n223 = Array Size(array=w254) -> (size(s)=w253:i32)
                n224 = case shown="4" w253 {
                  tunnel: ["콜 서비스 대기 중" "도착지로 이동 중 입니다." "콜  요청이 들어 왔습니다."] -> w252
                  frame 0, Default {
                  }
                  frame 2 {
                  }
                  frame 4 {
                  }
                }
              }
              frame True {
                n225 = Unbundle By Name(w283) -> ("d_lat"=w284:dbl, "d_lon"=w285:dbl)
                n226 = Unbundle By Name(w283) -> ("s_lat"=w313:dbl, "s_lon"=w312:dbl)
                n227 = global write "G_LCM.vi" "APP_GPS_DATA"(T11 {"hash"=3737605006820705978, "sys time"=0, "s_lat"=0.0, "s_lon"=0.0, "d_lat"=0.0, "d_lon"=0.0, "Message"=0} ("APP_GPS_DATA")) -> ()
                n228 = Build Array(w313, w312, 0.0 ("element")) -> (w310:dbl[])
                n229 = Build Array(w284, w285, 0.0 ("element")) -> (w287:dbl[])
                n230 = global read "G_NAV.vi" "ecef ref"() -> (w307:dbl[])
                n231 = global read "G_NAV.vi" "ecef ref"() -> (w290:dbl[])
                n232 = call "llh2XYZ.vi"("llh"=w310) -> ("DCM(ecef2lcc)"=w305:dbl[][], "ecef"=w308:dbl[])  [unwired: 7 in]
                n233 = call "llh2XYZ.vi"("llh"=w287) -> ("DCM(ecef2lcc)"=w292:dbl[][], "ecef"=w289:dbl[])  [unwired: 7 in]
                n234 = Subtract(x=w308, y=w307) -> (x-y=w309:dbl[])
                n235 = Subtract(x=w289, y=w290) -> (x-y=w288:dbl[])
                n236 = call-poly <vilib>:"Array To Matrix.vi"("Real 2D Array"=w305) -> ("Real Matrix"=w306:T13)
                n237 = call-poly <vilib>:"Array To Matrix.vi"("Real 2D Array"=w292) -> ("Real Matrix"=w291:T13)
                n238 = call-poly <vilib>:"Array To Matrix.vi"("Real 1D Array"=w309) -> ("Real Matrix (Column Vector)"=w304:T13)
                n239 = call-poly <vilib>:"Array To Matrix.vi"("Real 1D Array"=w288) -> ("Real Matrix (Column Vector)"=w293:T13)
                n240 = call-poly <vilib>:"Multiply.vi"("Real Matrix B"=w304, "Real Matrix A"=w306) -> ("A * B"=w301:T13)
                n241 = call-poly <vilib>:"Multiply.vi"("Real Matrix B"=w293, "Real Matrix A"=w291) -> ("A * B"=w296:T13)
                n242 = call-poly <vilib>:"Matrix To Array.vi"("Real Matrix"=w301) -> ("Real 2D Array"=w303:dbl[][])
                n243 = call-poly <vilib>:"Matrix To Array.vi"("Real Matrix"=w296) -> ("Real 2D Array"=w294:dbl[][])
                n244 = Index Array(array=w303, index (col)=0 ("disabled index (col)")) -> (element=w300:dbl[])  [unwired: 1 in]
                n245 = Index Array(array=w294, index (col)=0 ("disabled index (col)")) -> (element=w297:dbl[])  [unwired: 1 in]
                n246 = Index Array(array=w300, index #1=0 ("index")) -> (element #1=w282:dbl, element #2=w281:dbl)  [unwired: 1 in]
                n247 = Index Array(array=w297, index #1=0 ("index")) -> (element #1=w280:dbl, element #2=w279:dbl)  [unwired: 1 in]
                n248 = Build Array(w282, w281, w280, w279) -> (w278:dbl[])
              }
            }
            "Taxi" <- w226
            "String" <- w225
            n249 = Less?(x=w239, y=2025.0) -> (x < y?=w237:bool)
            n250 = case shown="True" w237 {
              tunnel: [_ w323] -> w251
              tunnel: [_ w320] -> w250
              tunnel: [_ w319] -> w249
              tunnel: [i32[] [0, 5, 0, 0] w318] -> w236
              frame False {
              }
              frame True {
                n251 = global read "G_LCM.vi" "APP_GPS_DATA"() -> (w321:T11)
                n252 = Unbundle By Name(w321) -> ("Message"=w322:i64)
                n253 = case shown="3" w322 {
                  tunnel: [_ TRUE _ _] -> w319
                  tunnel: [_ _ TRUE _] -> w320
                  tunnel: [_ _ _ TRUE] -> w323
                  tunnel: [i32[] [0, 5, 0, 0] i32[] [1, 5, 0, 0] i32[] [0, 2, 0, 0] i32[] [0, 5, 3, 0]] -> w318
                  frame 0, Default {
                  }
                  frame 1 {
                  }
                  frame 2 {
                  }
                  frame 3 {
                  }
                }
              }
            }
            "go" <- w251
            "left" <- w250
            "STOP" <- w249
            n254 = global write "G_VEH.vi" "E-STOP 2"(w249) -> ()
            n255 = for {
              tunnel: w236 -> [w315] mode=indexing
              tunnel: [w314] -> w235 mode=indexing
              n256 = local read "sign 2"() -> (w316:picture[])
              n257 = Index Array(array=w316, index=w315) -> (element=w314:picture)
            }
            "Array 3" <- w235
          }
          frame #4 {
            n258 = global read "G_VEH.vi" "candata"() -> (w352:T10)
            n259 = Unbundle By Name(w352) -> ("VS_des"=w332:dbl, "VS_can"=w345:dbl, "run"=w342:bool, "auto"=w343:bool, "Steer_input"=w336:dbl, "Steer_output"=w341:dbl)
            n260 = global read "G_VEH.vi" "VS_des"() -> (w333:dbl)
            n261 = global read "G_VEH.vi" "handle"() -> (w337:dbl)
            n262 = local read "replay"() -> (w334:bool)
            n263 = local read "replay"() -> (w338:bool)
            n264 = Not(x=w342) -> (.not. x?=w347:bool)
            n265 = Add(x=w341, y=0.0) -> (x+y=w339:dbl)
            n266 = Select(t=w336, s=w338, f=w337) -> (s? t:f=w335:dbl)
            n267 = Select(t=w332, s=w334, f=w333) -> (s? t:f=w331:dbl)
            n268 = Bundle(w347, "auto"=w343) -> (w349:cluster{bool, "auto":bool})  [unwired: 1 in]
            n269 = Boolean To (0,1)(Boolean=w349) -> (0, 1=→"Waveform Chart 4":cluster{i16, "auto":i16})
            n270 = Bundle("VS_des"=w332, "VS_can"=w345, "VS_des"=w331) -> (→"Gauge":T4)  [unwired: 1 in]
            n271 = Bundle("VS_des"=w332, "VS_can"=w345, "VS_des"=w331) -> (→"Waveform Chart 2":T4)  [unwired: 1 in]
            n272 = Bundle("Steer_input"=w336, w339, "handle"=w335) -> (w351:cluster{"Steer_input":dbl, dbl, "handle":dbl})  [unwired: 1 in]
            n273 = Negate(x=w351) -> (-x=→"Meter" →"Waveform Chart 3":cluster{"Steer_input":dbl, dbl, "handle":dbl})
          }
          frame #5 {
            n274 = global read "G_PATH.vi" "y origin"() -> (w360:dbl[])
            n275 = global read "G_PATH.vi" "x origin"() -> (w361:dbl[])
            n276 = global read "G_NAV.vi" "M6006"() -> (w365:T9)
            n277 = global read "G_VEH.vi" "xyhp"() -> (w359:T7)
            n278 = Unbundle By Name(w365) -> ("lcc[1]"=w366:dbl, "lcc[0]"=w367:dbl)
            n279 = local read "Taxi"() -> (w358:dbl[])
            n280 = Unbundle By Name(w359) -> ("x"=w363:dbl, "y"=w362:dbl)
            n281 = call "Convert to Dynamic Data6"("Array"=w361) -> ("Dynamic Data Type"=w369:dynamicdata)  [unwired: 3 in]
            n282 = call "Convert to Dynamic Data7"("Array"=w360) -> ("Dynamic Data Type"=w368:dynamicdata)  [unwired: 3 in]
            n283 = Array Size(array=w358) -> (size(s)=w357:i32)
            n284 = Merge Signals(w366, w369, w369, w363) -> (w355:dynamicdata)
            n285 = Merge Signals(w367, w368, w368, w362) -> (w353:dynamicdata)
            n286 = case shown="4" w357 {
              tunnel: [w371 w375 w389] -> w356
              tunnel: w355 -> [w371 w377 w390]
              tunnel: [w370 w372 w387] -> w354
              tunnel: w353 -> [w370 w374 w388]
              frame 0, Default {
              }
              frame 2 {
                n287 = local read "Taxi"() -> (w380:dbl[])
                n288 = Index Array(array=w380, index #1=1 ("index"), index #2=0 ("index")) -> (element #1=w376:dbl, element #2=w373:dbl)
                n289 = Merge Signals(w377, w376) -> (w375:dynamicdata)
                n290 = Merge Signals(w374, w373) -> (w372:dynamicdata)
              }
              frame 4 {
                n291 = local read "Taxi"() -> (w393:dbl[])
                n292 = Index Array(array=w393, index #1=1 ("index"), index #2=3 ("index"), index #3=0 ("index"), index #4=2 ("index")) -> (element #1=w384:dbl, element #2=w383:dbl, element #3=w382:dbl, element #4=w381:dbl)
                n293 = Merge Signals(w390, w384, w383) -> (w389:dynamicdata)
                n294 = Merge Signals(w388, w382, w381) -> (w387:dynamicdata)
              }
            }
            n295 = call "GRAPH"("Y Input"=w354, "X Input"=w356) -> ("XY Graph"=→"XY Graph 2":cluster{"Y":dbl[], "Y":dbl[]}[])  [unwired: 3 in, 6 out]
          }
        }
      }
    }
  }
  n296 = flat-sequence {
    frame #0 {
      # "1. Alogorithm\n2. Make & Laod path"
    }
    frame #1 {
      w394 = FALSE ("lane update")
      w399 = FALSE ("Make WPT")
      n297 = Current VI's Path() -> (path=w398:path)
      n298 = global write "G_VEH.vi" "handle"(0.0 ("handle")) -> ()
      n299 = local write "Make WPT"(w399) -> ()
      n300 = local write "Load WPT"(w399) -> ()
      n301 = local write "lane"(w394) -> ()
      n302 = Strip Path(path=w398) -> (stripped path=w397:path)  [unwired: 1 out]
      n303 = local write "lane keep"(w394) -> ()
      n304 = global write "G_DATA.vi" "path"(w397) -> ()
      n305 = local write "x"(0.0 ("x")) -> ()
    }
    frame #2 {
      n306 = while {
        stop <- FALSE stop-if-true
        n307 = flat-sequence {
          frame #0 {
            n308 = Wait Until Next ms Multiple(millisecond multiple=u32 10 ("milliseconds to wait")) -> (millisecond timer value=w401:u32)
            n309 = feedback #6() -> (w403:u32)  [unwired: 1 in]
            n310 = feedback-in #6(w401) -> ()
            n311 = Subtract(x=w401, y=w403) -> (x-y=→"path":u32)
          }
          frame #1 {
            n312 = case shown="False" "Make WPT" {
              frame False {
                n313 = case shown="False" "Load WPT" {
                  frame False {
                    n314 = disable-structure shown="Enabled" {
                      frame Enabled {
                        n315 = flat-sequence {
                          tunnel: [w529] -> w407
                          tunnel: w407 -> [w545]
                          frame #0 {
                            n316 = local read "x"() -> (w412:dbl)
                            n317 = global read "G_SEN.vi" "M_lane_update"() -> (w413:bool)
                            n318 = Equal To 0?(x=w412) -> (x = 0?=w411:bool)
                            n319 = Or(x=w411, y="lane") -> (x .or. y?=w410:bool)
                            n320 = And(x=w413, y=w410) -> (x .and. y?=w414:bool)
                            n321 = case shown="True" w414 {
                              tunnel: "vehicel width" -> [_ w417]
                              tunnel: "lane" -> [_ _]
                              frame False {
                              }
                              frame True {
                                n322 = case shown="True" TRUE {
                                tunnel: w417 -> [w419 _]
                                tunnel: [w418 w524] -> w416
                                frame False {
                                n323 = flat-sequence {
                                tunnel: [w422] -> w420
                                tunnel: w419 -> [w421]
                                tunnel: w420 -> [w519]
                                tunnel: [w517] -> w418
                                frame #0 {
                                n324 = Add(x=w421, y=1.0) -> (x+y=w433:dbl)
                                n325 = global read "G_SEN.vi" "Lane_L_M"() -> (w439:dbl[])
                                n326 = global read "G_SEN.vi" "Lane_R_M"() -> (w438:dbl[])
                                n327 = Index Array(array=w439, index #1=3 ("index"), index #2=0 ("index")) -> (element #1=w424:dbl, element #2=w429:dbl)
                                n328 = Index Array(array=w438, index #1=0 ("index"), index #2=3 ("index")) -> (element #1=w437:dbl, element #2=w423:dbl)
                                n329 = Greater Or Equal?(x=w429, y=0.8) -> (x >= y?=w428:bool)
                                n330 = Greater Or Equal?(x=w437, y=0.8) -> (x >= y?=w427:bool)
                                n331 = And(x=w428, y=w427) -> (x .and. y?=w426:bool)
                                n332 = Multiply(x=w433, y=0.5) -> (x*y=w431:dbl)
                                n333 = case shown="True" w426 {
                                tunnel: w431 -> [w442 w491]
                                tunnel: w424 -> [_ w493]
                                tunnel: w423 -> [_ w492]
                                tunnel: [w443 w489] -> w422
                                frame False {
                                n334 = global read "G_SEN.vi" "Lane_L_M"() -> (w447:dbl[])
                                n335 = Index Array(array=w447, index #1=3 ("index"), index #2=0 ("index")) -> (element #1=w444:dbl, element #2=w449:dbl)
                                n336 = Greater Or Equal?(x=w449, y=0.8) -> (x >= y?=w445:bool)
                                n337 = case shown="True" w445 {
                                tunnel: w444 -> [_ w484]
                                tunnel: w442 -> [w452 w483]
                                tunnel: [w451 w479] -> w443
                                frame False {
                                n338 = global read "G_SEN.vi" "Lane_R_M"() -> (w456:dbl[])
                                n339 = Index Array(array=w456, index #1=0 ("index"), index #2=3 ("index")) -> (element #1=w457:dbl, element #2=w453:dbl)
                                n340 = Greater Or Equal?(x=w457, y=0.8) -> (x >= y?=w454:bool)
                                n341 = case shown="True" w454 {
                                tunnel: w453 -> [_ w473]
                                tunnel: w452 -> [_ w472]
                                tunnel: [w460 w465] -> w451
                                frame False {
                                n342 = global read "G_SEN.vi" "Lane_C_M"() -> (w462:dbl[])
                                n343 = Index Array(array=w462, index=3) -> (element=w460:dbl)
                                }
                                frame True {
                                n344 = Subtract(x=w473, y=w472) -> (x-y=w471:dbl)
                                n345 = global read "G_SEN.vi" "Lane_C_M"() -> (w470:dbl[])
                                n346 = Greater Than 0?(x=w471) -> (x > 0?=w467:bool)
                                n347 = Index Array(array=w470, index=3) -> (element=w464:dbl)
                                n348 = Less Than 0?(x=w464) -> (x < 0?=w468:bool)
                                n349 = local read "lane_shift"() -> (w463:dbl)
                                n350 = And(x=w467, y=w468) -> (x .and. y?=w466:bool)
                                n351 = Select(t=w463, s=w466, f=w464) -> (s? t:f=w465:dbl)
                                }
                                }
                                }
                                frame True {
                                n352 = Add(x=w484, y=w483) -> (x+y=w482:dbl)
                                n353 = global read "G_SEN.vi" "Lane_C_M"() -> (w481:dbl[])
                                n354 = Less Than 0?(x=w482) -> (x < 0?=w477:bool)
                                n355 = Index Array(array=w481, index=3) -> (element=w475:dbl)
                                n356 = Greater Than 0?(x=w475) -> (x > 0?=w478:bool)
                                n357 = local read "lane_shift"() -> (w474:dbl)
                                n358 = And(x=w477, y=w478) -> (x .and. y?=w476:bool)
                                n359 = Select(t=w474, s=w476, f=w475) -> (s? t:f=w479:dbl)
                                }
                                }
                                }
                                frame True {
                                n360 = Add(x=w493, y=w491) -> (x+y=w486:dbl)
                                n361 = Subtract(x=w492, y=w491) -> (x-y=w485:dbl)
                                n362 = Less Than 0?(x=w486) -> (x < 0?=w488:bool)
                                n363 = Greater Than 0?(x=w485) -> (x > 0?=w487:bool)
                                n364 = Not Equal?(x=w488, y=w487) -> (x != y?=w490:bool)
                                n365 = case shown="True" w490 {
                                tunnel: [w496 w502] -> w489
                                tunnel: w488 -> [w501 _]
                                tunnel: w487 -> [w500 w509]
                                tunnel: w486 -> [_ w508]
                                tunnel: w485 -> [_ w507]
                                frame False {
                                n366 = And(x=w501, y=w500) -> (x .and. y?=w497:bool)
                                n367 = global read "G_SEN.vi" "Lane_C_M"() -> (w498:dbl[])
                                n368 = local read "lane_shift"() -> (w495:dbl)
                                n369 = Index Array(array=w498, index=3) -> (element=w494:dbl)
                                n370 = Select(t=w495, s=w497, f=w494) -> (s? t:f=w496:dbl)
                                }
                                frame True {
                                n371 = Select(t=w508, s=w509, f=w507) -> (s? t:f=w506:dbl)
                                n372 = global read "G_SEN.vi" "Lane_C_M"() -> (w510:dbl[])
                                n373 = Index Array(array=w510, index=3) -> (element=w505:dbl)
                                n374 = Add(x=w505, y=w506) -> (x+y=w504:dbl)
                                n375 = Multiply(x=w504, y=0.5) -> (x*y=w502:dbl)
                                }
                                }
                                }
                                }
                                }
                                frame #1 {
                                n376 = global read "G_SEN.vi" "Lane_C_M"() -> (w523:dbl[])
                                n377 = local read "lane_shift"() -> (w515:dbl)
                                n378 = Index Array(array=w523, index=3) -> (element=w516:dbl)
                                n379 = Add(x=w516, y=w515) -> (x+y=w514:dbl)
                                n380 = In Range and Coerce(upper limit=0.5, x=w516, lower limit=-0.5) -> (In Range?=w518:bool)  [unwired: 1 out]
                                n381 = Multiply(x=0.5, y=w514) -> (x*y=w512:dbl)
                                n382 = Select(t=w519, s=w518, f=w512) -> (s? t:f=w517:dbl)
                                }
                                }
                                }
                                frame True {
                                n383 = disable-structure shown="Enabled" {
                                frame Disabled {
                                n384 = local write "lane"(FALSE ("lane update")) -> ()
                                n385 = local write "x"(0.0 ("x")) -> ()
                                }
                                frame Enabled {
                                }
                                }
                                n386 = global read "G_SEN.vi" "Lane_C_M"() -> (w526:dbl[])
                                n387 = Index Array(array=w526, index=3) -> (element=w524:dbl)
                                }
                                }
                                "lane_shift" <- w416
                              }
                            }
                          }
                          frame #1 {
                            n388 = local read "vehicel width"() -> (w544:dbl)
                            n389 = call "obstest.vi"("vehicle width"=w544) -> ("out"=w539:dbl)  [unwired: 9 in, 1 out]
                            "obs shift" <- w539
                            n390 = local read "lane_shift"() -> (w537:dbl)
                            n391 = In Range and Coerce(upper limit=0.15, x=w539, lower limit=-0.15) -> (coerced(x)=w541:dbl)  [unwired: 1 out]
                            n392 = Multiply(x="x", y=0.25) -> (x*y=w530:dbl)
                            n393 = Compound Arithmetic op=ADD(w541, w537, w530) -> (w533:dbl)
                            n394 = Decrement(x="Shift LPF gain") -> (x-1=w534:dbl)
                            n395 = feedback #7(w533) -> (w532:dbl)
                            n396 = Multiply(x=w532, y="Shift LPF gain") -> (x*y=w535:dbl)
                            n397 = Multiply(x=w534, y=w533) -> (x*y=w536:dbl)
                            n398 = Subtract(x=w535, y=w536) -> (x-y=w529:dbl)
                            n399 = feedback-in #7(w529) -> ()
                          }
                          frame #2 {
                            n400 = case shown="True" "lane keep" {
                              frame False {
                              }
                              frame True {
                                n401 = local write "x"(0.0 ("x")) -> ()
                              }
                            }
                            n402 = call "tracking1.vi"("lane keep"="lane keep", "xt"=w545) -> ("handle"=w546:dbl)  [unwired: 8 in, 1 out]
                            n403 = flat-sequence {
                              tunnel: w546 -> [w550]
                              frame #0 {
                                n404 = disable-structure shown="Enabled" {
                                disable-tunnel: w550 -> [w554 w568]
                                disable-tunnel: [w555 "Steering gain"] -> w549
                                disable-tunnel: [w554 w568] -> w548
                                frame Enabled {
                                w557 = 20.0 ("y")
                                n405 = Absolute Value(x=w554) -> (abs(x)=w558:dbl)
                                n406 = Greater?(x=w558, y=w557) -> (0:w559:bool)
                                n407 = case shown="True" w559 {
                                tunnel: w558 -> [_ w567]
                                tunnel: w557 -> [_ w566]
                                tunnel: [_ w560] -> w556
                                frame False {
                                }
                                frame True {
                                n408 = Subtract(x=w567, y=w566) -> (x-y=w565:dbl)
                                n409 = Multiply(x=w565, y=0.01) -> (x*y=w563:dbl)
                                n410 = In Range and Coerce(upper limit=0.1, x=w563, lower limit=0.0) -> (coerced(x)=w560:dbl)  [unwired: 1 out]
                                }
                                }
                                n411 = Increment(x=w556) -> (x+1=w555:dbl)
                                }
                                frame Disabled {
                                }
                                }
                                n412 = Multiply(x=w548, y=w549) -> (x*y=w551:dbl)
                                n413 = disable-structure shown="Enabled" {
                                disable-tunnel: [w579 w580] -> w552
                                disable-tunnel: w551 -> [w576 w580]
                                frame Disabled {
                                n414 = Decrement(x="Steering LPF gain") -> (x-1=w577:dbl)
                                n415 = feedback #8(w576) -> (w578:dbl)
                                n416 = Multiply(x=w578, y="Steering LPF gain") -> (x*y=w574:dbl)
                                n417 = Multiply(x=w577, y=w576) -> (x*y=w575:dbl)
                                n418 = Subtract(x=w574, y=w575) -> (x-y=w579:dbl)
                                n419 = feedback-in #8(w579) -> ()
                                }
                                frame Enabled {
                                }
                                }
                                n420 = disable-structure shown="Enabled" {
                                disable-tunnel: [w571 w572] -> w553
                                disable-tunnel: w552 -> [w570 w572]
                                frame Disabled {
                                n421 = feedback #9(w570) -> (w571:dbl)
                                n422 = feedback-in #9(w570) -> ()
                                }
                                frame Enabled {
                                }
                                }
                                n423 = global write "G_VEH.vi" "handle"(w553) -> ()
                              }
                            }
                          }
                        }
                      }
                      frame Disabled {
                      }
                    }
                  }
                  frame True {
                    n424 = flat-sequence {
                      frame #0 {
                        w583 = FALSE ("X Scale.Loose Fit")
                        w582 = u8 0 ("X Scale.Scale Fit")
                        n425 = call "initvar.vi"() -> ()  [unwired: 12 in]
                        n426 = property on="XY Graph" class="XYGraph (strict)"("XScale.ScaleFit"=w582, "YScale.ScaleFit"=w582, "XScale.LooseFit"=w583, "YScale.LooseFit"=w583) -> ()  [unwired: 2 in, 2 out]
                      }
                      frame #1 {
                        n427 = global read "G_VEH.vi" "Location"() -> (w584:i32)
                        n428 = Bundle("Minimum"=-5.0, "Minimum"=37.3, "Minimum"=10.0, "Minimum"=1.0, "Minimum"=-20.0) -> (w590:T14)  [unwired: 1 in]
                        n429 = Bundle("Minimum"=-22.6, "Minimum"=22.6, "Minimum"=10.0, "Minimum"=1.0, "Minimum"=-20.0) -> (w597:T14)  [unwired: 1 in]
                        n430 = call "getecefdcmref.vi"("map"=w584) -> ("XYZ"=w585:dbl[])  [unwired: 10 in, 4 out]
                        n431 = property on="XY Graph" class="XYGraph (strict)"("YScale.Range"=w590) -> ()  [unwired: 2 in, 2 out]
                        n432 = property on="XY Graph" class="XYGraph (strict)"("XScale.Range"=w597) -> ()  [unwired: 2 in, 2 out]
                        n433 = global write "G_NAV.vi" "ecef ref"(w585) -> ()
                      }
                      frame #2 {
                        n434 = global read "G_DATA.vi" "path"() -> (w601:path)
                        n435 = Build Path(base path=w601, name or relative path="wpt") -> (appended path=w599:path)
                        n436 = call "Read From Measurement File2"("Filename"=w599, "Reset"=TRUE) -> ("error out"=w603:errorcluster, "Filename Out"=w598:path, "Signals"=w605:dynamicdata)  [unwired: 4 in, 3 out]
                        n437 = Unbundle By Name(w603) -> ("status"=w602:bool)
                        n438 = case shown="False" w602 {
                          tunnel: w605 -> [w607 _]
                          tunnel: w598 -> [w606 _]
                          frame False {
                            n439 = call "Convert from Dynamic Data2"("Dynamic Data Type"=w607) -> ("Array"=w609:dbl[][])  [unwired: 3 in]
                            n440 = Empty Array?(array=w609) -> (empty?=w608:bool)
                            n441 = case shown="False" w608 {
                              tunnel: w609 -> [w611 _]
                              tunnel: w606 -> [w610 _]
                              frame False {
                                n442 = call "path_ini_new.vi"("Filename Out"=w610, "WPT"=w611) -> ()  [unwired: 10 in]
                              }
                              frame True {
                                w612 = dbl[][] [] ("path_updated")
                                n443 = global write "G_PATH.vi" "path"(w612) -> ()
                                n444 = global write "G_PATH.vi" "path_very_origin"(w612) -> ()
                                n445 = global write "G_PATH.vi" "path_origin"(w612) -> ()
                              }
                            }
                          }
                          frame True {
                            w613 = dbl[][] [] ("path_updated")
                            n446 = global write "G_PATH.vi" "path"(w613) -> ()
                            n447 = global write "G_PATH.vi" "path_very_origin"(w613) -> ()
                            n448 = global write "G_PATH.vi" "path_origin"(w613) -> ()
                          }
                        }
                      }
                      frame #3 {
                        w614 = T15 [] ("Missions_origin")
                        n449 = global read "G_VEH.vi" "Location"() -> (w615:i32)
                        n450 = local write "Load WPT"(FALSE ("Load WPT")) -> ()
                        n451 = global write "G_PATH.vi" "Missions_origin"(w614) -> ()
                        n452 = global write "G_PATH.vi" "Missions"(w614) -> ()
                        n453 = call "mapconf.vi"("Location"=w615) -> ("y"=w617:cluster{dbl, dbl, "y":dbl, "y":dbl, dbl}, "x"=w618:cluster{dbl, dbl, "y":dbl, "y":dbl, dbl}, "new picture"=w619:picture)  [unwired: 8 in]
                        n454 = property on="XY Graph 2" class="XYGraph (strict)"("PlotImages.Back"=w619) -> ()  [unwired: 2 in, 2 out]
                        n455 = property on="XY Graph 2" class="XYGraph (strict)"("XScale.Range"=w618, "YScale.Range"=w617) -> ()  [unwired: 2 in, 2 out]
                      }
                    }
                  }
                }
              }
              frame True {
                n456 = flat-sequence {
                  tunnel: [w624] -> w620
                  tunnel: w620 -> [w713]
                  frame #0 {
                    w621 = 0.0
                    n457 = global write "G_VEH.vi" "handle"(w621) -> ()
                    n458 = global write "G_VEH.vi" "VS_des"(w621) -> ()
                  }
                  frame #1 {
                    n459 = local read "Make WPT"() -> (w623:bool)
                    n460 = global read "G_VEH.vi" "Location"() -> (w622:i32)
                    n461 = Initialize Array(0.0 ("element"), 7 ("dimension size"), 1 ("dimension size")) -> (w625:dbl[][])
                    n462 = while {
                      shift-right: [w630] -> w624
                      shift-left: w625 -> [w632]
                      shift-right: [FALSE] -> _
                      shift-left: w623 -> [w633]
                      tunnel: w622 -> [w629]
                      stop <- w635 stop-if-true
                      n463 = flat-sequence {
                        tunnel: [w645] -> w631
                        tunnel: w629 -> [w638]
                        frame #0 {
                          n464 = global read "G_NAV.vi" "GPS_status"() -> (w637:T16)
                          n465 = disable-structure shown="Enabled" {
                            disable-tunnel: [w656 w660] -> w648
                            disable-tunnel: [w655 w659] -> w647
                            disable-tunnel: [w649 w658] -> w646
                            disable-tunnel: w637 -> [w654 w668]
                            disable-tunnel: [w653 w667] -> w644
                            disable-tunnel: [w652 w666] -> w643
                            disable-tunnel: [w649 w665] -> w642
                            disable-tunnel: w638 -> [_ w664]
                            frame Enabled {
                              n466 = Unbundle By Name(w654) -> ("lat"=w653:dbl, "lon"=w652:dbl, "hgt"=w649:dbl)
                              n467 = global read "G_NAV.vi" "M6006"() -> (w657:T9)
                              n468 = Unbundle By Name(w657) -> ("lcc[0]"=w651:dbl, "lcc[1]"=w650:dbl)
                              n469 = To Double Precision Float(number=w651) -> (double precision float=w656:dbl)
                              n470 = To Double Precision Float(number=w650) -> (double precision float=w655:dbl)
                            }
                            frame Disabled {
                              n471 = Unbundle By Name(w668) -> ("lat"=w667:dbl, "lon"=w666:dbl, "hgt"=w665:dbl)
                              n472 = call "getecefdcmref.vi"("map"=w664) -> ("XYZ"=w663:dbl[])  [unwired: 10 in, 4 out]
                              n473 = call "llh2lcc.vi"("ecef ref"=w663, "hgt"=w665, "lon"=w666, "lat"=w667) -> ("lcc"=w662:dbl[])  [unwired: 7 in]
                              n474 = Index Array(array=w662, index #1=0 ("index")) -> (element #1=w660:dbl, element #2=w659:dbl, element #3=w658:dbl)  [unwired: 2 in]
                            }
                          }
                          n475 = To Double Precision Float(number=w638) -> (double precision float=w639:dbl)
                          n476 = global read "G_VEH.vi" "candata"() -> (w641:T10)
                          n477 = Unbundle By Name(w641) -> ("VS_can"=w640:dbl)
                          n478 = Build Array(w644, w643, w642, w648, w647, w646, w640, w639) -> (w645:dbl[])
                        }
                      }
                      n479 = local read "Make WPT"() -> (w636:bool)
                      n480 = Not(x=w636) -> (.not. x?=w635:bool)
                      n481 = case shown="False" w633 {
                        tunnel: w632 -> [w683 w700]
                        tunnel: w631 -> [w682 w698]
                        tunnel: [w681 w697] -> w630
                        frame False {
                          n482 = Array Size(array=w683) -> (size(s)=w691:i32[])
                          n483 = Index Array(array=w682, index #1=3 ("index"), index #2=4 ("index")) -> (element #1=w677:dbl, element #2=w675:dbl)
                          n484 = Index Array(array=w691, index=1) -> (element=w680:i32)
                          n485 = Decrement(x=w680) -> (x-1=w679:i32)
                          n486 = Index Array(array=w683, index (col)=w679) -> (element=w687:dbl[])  [unwired: 1 in]
                          n487 = Index Array(array=w687, index #1=3 ("index"), index #2=4 ("index")) -> (element #1=w678:dbl, element #2=w676:dbl)
                          n488 = Subtract(x=w678, y=w677) -> (x-y=w674:dbl)
                          n489 = Subtract(x=w676, y=w675) -> (x-y=w673:dbl)
                          n490 = Square(x=w674) -> (x^2=w672:dbl)
                          n491 = Square(x=w673) -> (x^2=w671:dbl)
                          n492 = Add(x=w672, y=w671) -> (x+y=w670:dbl)
                          n493 = Greater Or Equal?(x=w670, y=0.25) -> (x >= y?=w684:bool)
                          n494 = case shown="True" w684 {
                            tunnel: w683 -> [w692 w696]
                            tunnel: w680 -> [_ w693]
                            tunnel: w682 -> [_ w695]
                            tunnel: [w692 w694] -> w681
                            frame False {
                            }
                            frame True {
                              n495 = Insert Into Array(array=w696, index (col)=w693, new element=w695) -> (w694:dbl[][])  [unwired: 1 in]
                            }
                          }
                        }
                        frame True {
                          n496 = Replace Array Subset(array=w700, new element=w698, index (col)=0 ("disabled index (col)")) -> (w697:dbl[][])  [unwired: 1 in]
                        }
                      }
                    }
                  }
                  frame #2 {
                    n497 = call "Convert to Dynamic Data"("2D Array"=w713) -> ("Dynamic Data Type"=w714:dynamicdata)  [unwired: 3 in]
                    n498 = global read "G_VEH.vi" "Location"() -> (w710:i32)
                    n499 = case shown="9" w710 {
                      tunnel: ["" ("String") "Hyundai" ("String") "KAIST" ("String") "AJOU" ("String") "MUNJI" ("String") "Airforce" ("String") "CAR" ("String") "KATRI" ("String") _ "coex" ("String")] -> w709
                      frame 0, Default {
                      }
                      frame 1 {
                      }
                      frame 2 {
                      }
                      frame 3 {
                      }
                      frame 4 {
                      }
                      frame 5 {
                      }
                      frame 6 {
                      }
                      frame 7 {
                      }
                      frame 8 {
                      }
                      frame 9 {
                      }
                    }
                    n500 = Get Date/Time In Seconds() -> (seconds since 1Jan1904=w711:timestamp)
                    n501 = Format Date/Time String(time format string (%c)="%2y%2m%2d%2H%2M", seconds (now)=w711) -> (date/time string=w707:string)  [unwired: 1 in]
                    n502 = global read "G_DATA.vi" "path"() -> (w705:path)
                    n503 = Build Path(base path=w705, name or relative path="wpt") -> (appended path=w703:path)
                    n504 = Concatenate Strings(w707, "_" ("string"), w709, ".lvm" ("string")) -> (w702:string)
                    n505 = Build Path(base path=w703, name or relative path=w702) -> (appended path=w701:path)
                    n506 = call "save wpt"("Signals"=w714, "Reset"=TRUE, "Filename"=w701) -> ()  [unwired: 14 in, 3 out]
                  }
                }
              }
            }
          }
        }
      }
    }
  }
  n507 = flat-sequence {
    frame #0 {
      # "Sensor paser"
    }
    frame #1 {
      w726 = dbl[][] [] ("sensor_car")
      w727 = dbl[][] [] ("sensor_lane_log")
      n508 = disable-structure shown="Enabled" {
        disable-tunnel: [dbl[][] array18932x2[37864 elements] ("all rows") _] -> w725
        frame Disabled {
        }
        frame Enabled {
        }
      }
      n509 = local write "Log"(FALSE ("obs")) -> ()
      n510 = global write "G_SEN.vi" "data"(w726) -> ()
      n511 = global write "G_SEN.vi" "sensor_lane_log"(w727) -> ()
      n512 = global write "G_SEN.vi" "sensor_obs_log"(w727) -> ()
      n513 = global write "G_SEN.vi" "sensor_etc"(w726) -> ()
      n514 = global write "G_SEN.vi" "sensor_lane"(w726) -> ()
      n515 = global write "G_SEN.vi" "sensor_obs"(w726) -> ()
      n516 = global write "G_SEN.vi" "map_lane"(w725) -> ()
    }
    frame #2 {
      n517 = while {
        stop <- FALSE stop-if-true
        n518 = flat-sequence {
          frame #0 {
            n519 = Wait Until Next ms Multiple(millisecond multiple=u32 10 ("milliseconds to wait")) -> (millisecond timer value=w731:u32)
            n520 = feedback #10() -> (w733:u32)  [unwired: 1 in]
            n521 = feedback-in #10(w731) -> ()
            n522 = Subtract(x=w731, y=w733) -> (x-y=→"sensor":u32)
          }
          frame #1 {
            n523 = disable-structure shown="Enabled" {
              frame Enabled {
                n524 = call "mobileyepaser.vi"() -> ()  [unwired: 11 in, 1 out]
                n525 = call "mobileyelanepaser4.vi"("count hold"=u64 15, "thresh  c"=0.5, "thresh  b"=0.06 ("thresh 2"), "thresh r"=0.009 ("y")) -> ()  [unwired: 4 in, 4 out]
              }
              frame Disabled {
              }
            }
          }
          frame #2 {
            n526 = disable-structure shown="Disabled" {
              frame Disabled {
                n527 = call "velodynepaser.vi"() -> ()  [unwired: 10 in, 2 out]
              }
              frame Enabled {
              }
            }
          }
          frame #3 {
            w741 = TRUE ("Sensor [F12]")
            n528 = global read "G_SEN.vi" "M_lane_update"() -> (→"update":bool)
            n529 = call "Ibeopaser.vi"("theta"=-2.5, "Hide Transparent"=w741, "Sensor [F12]"=w741) -> ("x_sensor"=w745:T7, "etc"=w743:dbl[][], "lane"=w744:dbl[][], "obs"=w746:dbl[][], "update"=w742:bool)  [unwired: 4 in]
            n530 = case shown="True" w742 {
              tunnel: w746 -> [_ w751]
              tunnel: w745 -> [_ w752]
              tunnel: w744 -> [_ w748]
              tunnel: w743 -> [_ w749]
              frame False {
              }
              frame True {
                n531 = disable-structure shown="Enabled" {
                  disable-tunnel: w751 -> [w757 w759]
                  disable-tunnel: [w756 w759] -> w750
                  disable-tunnel: w749 -> [w755 _]
                  disable-tunnel: w748 -> [w754 w758]
                  disable-tunnel: [w753 w758] -> w747
                  frame Disabled {
                    n532 = call "test3.vi"("sensor_all"=w755, "sensor_lane"=w754, "sensor_obs"=w757) -> ("lane"=w753:dbl[][], "obs"=w756:dbl[][])  [unwired: 6 in, 1 out]
                  }
                  frame Enabled {
                  }
                }
                n533 = global write "G_VEH.vi" "xsensor"(w752) -> ()
                n534 = global write "G_SEN.vi" "sensor_obs"(w750) -> ()
                n535 = global write "G_SEN.vi" "sensor_lane"(w747) -> ()
              }
            }
          }
          frame #4 {
            n536 = case shown="True" "Log" {
              frame False {
                n537 = global write "G_SEN.vi" "sensor_obs_log"(dbl[][] [] ("sensor_obs_log")) -> ()
              }
              frame True {
                n538 = global read "G_VEH.vi" "candata"() -> (w763:T10)
                n539 = Unbundle By Name(w763) -> ("VS_can"=w764:dbl)
                n540 = Not Equal To 0?(x=w764) -> (x != 0?=w762:bool)
                n541 = case shown="True" w762 {
                  frame False {
                  }
                  frame True {
                    n542 = global read "G_SEN.vi" "sensor_obs_log"() -> (w766:dbl[][])
                    n543 = global read "G_SEN.vi" "sensor_obs"() -> (w767:dbl[][])
                    n544 = call "sensor_log2.vi"("xmax"=8.0, "range^2"=16.0, "xmin"=-5.0, "FF"=0.93 ("t"), "ymin"=0.0, "ymax"=20.0, "sensor_log"=w766, "sensor_obs"=w767) -> ("sensor_log 2"=w765:dbl[][])  [unwired: 2 in, 1 out]
                    n545 = global write "G_SEN.vi" "sensor_obs_log"(w765) -> ()
                  }
                }
              }
            }
          }
          frame #5 {
            n546 = disable-structure shown="Enabled" {
              frame Enabled {
                n547 = global read "G_VEH.vi" "candata"() -> (w780:T10)
                n548 = global read "G_VEH.vi" "sys time"() -> (w775:i64)
                n549 = Unbundle By Name(w780) -> ("VS_can"=w781:dbl)
                n550 = feedback-in #11(w775) -> ()
                n551 = feedback #11(i64 0 ("sys time")) -> (w779:i64)
                n552 = Not Equal To 0?(x=w781) -> (x != 0?=w777:bool)
                n553 = Greater?(x=w775, y=w779) -> (0:w778:bool)
                n554 = And(x=w777, y=w778) -> (x .and. y?=w776:bool)
                n555 = case shown="True" w776 {
                  frame False {
                  }
                  frame True {
                    n556 = flat-sequence {
                      tunnel: [w783] -> w782
                      tunnel: w782 -> [w801]
                      frame #0 {
                        n557 = disable-structure shown="Enabled" {
                          disable-tunnel: [50.0 ("ymax") 10000.0 ("ymax")] -> w788
                          disable-tunnel: [-3.5 ("ymin") -10000.0 ("ymin")] -> w787
                          disable-tunnel: [-6.0 ("xmin") -10000.0 ("xmin")] -> w786
                          disable-tunnel: [10.0 ("xmin") 10000.0 ("xmax")] -> w785
                          frame Enabled {
                          }
                          frame Disabled {
                          }
                        }
                        n558 = global read "G_SEN.vi" "sensor_lane_log"() -> (w792:dbl[][])
                        n559 = global read "G_SEN.vi" "sensor_lane"() -> (w791:dbl[][])
                        n560 = call "sensor_log2.vi"("xmax"=w785, "range^2"=0.0, "xmin"=w786, "FF"=1.0, "ymin"=w787, "ymax"=w788, "sensor_log"=w792, "sensor_obs"=w791) -> ("sensor_log_body"=w783:dbl[][], "sensor_log 2"=w784:dbl[][])  [unwired: 2 in]
                        n561 = global write "G_SEN.vi" "sensor_lane_log"(w784) -> ()
                      }
                      frame #1 {
                        n562 = disable-structure shown="Enabled" {
                          disable-tunnel: w801 -> [w802 _]
                          frame Disabled {
                            n563 = call "lane_test1.vi"("lane_body"=w802) -> ()  [unwired: 11 in]
                          }
                          frame Enabled {
                          }
                        }
                      }
                    }
                  }
                }
              }
              frame Disabled {
              }
            }
          }
        }
      }
    }
  }
